vi "Send 2D image to FPGA.vi"(7 "picture":picture, 8 "error in":errorcluster, 11 "FPGA VI Reference Out":T1) -> (0 "error out":errorcluster, 3 "FPGA VI Reference Out 2":T1)   [LabVIEW 2019]
uses:
  TypeDefs/FPGA Reference.ctl
  <vilib>/Utility/error.llb/Error Cluster From Error Code.vi
  <vilib>/rvi/errors/niLvFpgaAdjustHostInterfaceError.vi
  <vilib>/rvi/interface/nirviMethod/nirviMethod.xnode
  FPGA Bitfiles/adafruitlcdsom_FPGATarget_FPGAMain_K7l+4zj6vFY.lvbitx
  FPGA Main.vi
  <vilib>/FPGAPlugInAG/sbRIO-9651/niLvFpga_WriteFifo_sbRIO-9651.vi
  <vilib>/rvi/errors/niLvFpgaMergeErrorWithErrorCode.vi
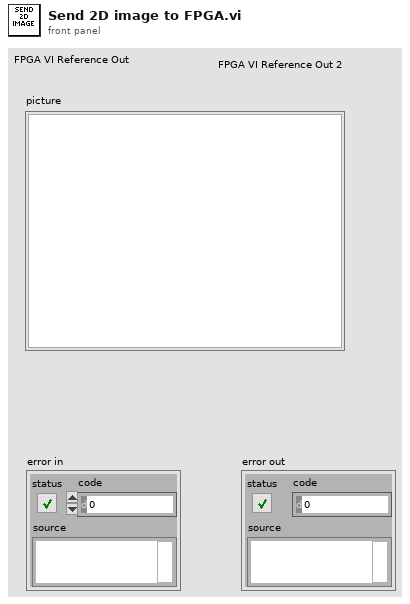
[diagram p1: front panel]
types:
  T1 = typedef "FPGA Reference.ctl" = refnum<k20>
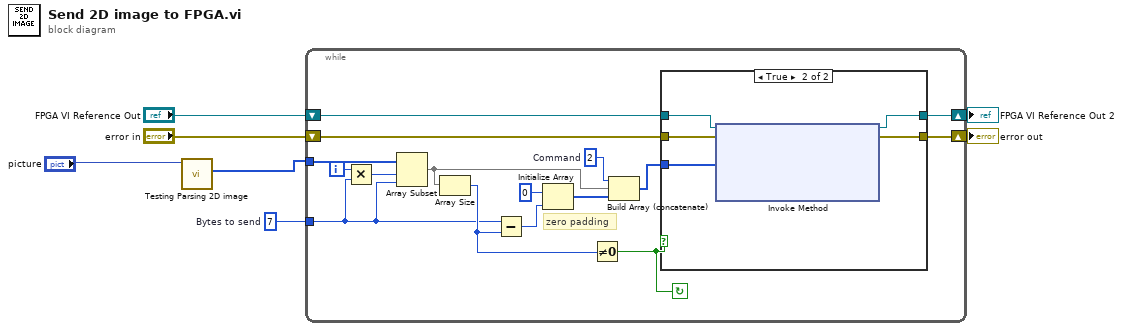
[diagram p0: block diagram]
diagram:
  w4 = 7  # Bytes to send
  n1 = call "Testing Parsing 2D image.vi"("2D Picture"="picture") -> ("output array"=w1:u16[])  [unwired: 9 in, 1 out]
  n2 = while {
    shift-right: [w22] -> w6
    shift-left: "FPGA VI Reference Out" -> [w23]
    shift-right: [w21] -> w5
    shift-left: "error in" -> [w20]
    tunnel: w1 -> [w17]
    tunnel: w4 -> [w8]
    i -> [w16]
    stop <- w11 continue-if-true
    w19 = u16 2  # Command
    # "zero padding"
    n3 = Multiply(x=w16, y=w8) -> (x*y=w15:i32)
    n4 = Array Subset(array=w17, index=w15, length=w8) -> (w14:u16[])
    n5 = Array Size(array=w14) -> (size(s)=w10:i32)
    n6 = Subtract(x=w8, y=w10) -> (x-y=w9:i32)
    n7 = Initialize Array(u16 0 ("X"), w9) -> (w12:u16[])
    n8 = Not Equal To 0?(x=w10) -> (x != 0?=w11:bool)
    n9 = Build Array (concatenate)(w19, w14, w12) -> (w18:u16[])
    n10 = case shown="True" w11 {
      tunnel: w23 -> [w25 w30]
      tunnel: [w25 w29] -> w22
      tunnel: [w24 w28] -> w21
      tunnel: w20 -> [w24 w27]
      tunnel: w18 -> [_ w26]
      frame False {
      }
      frame True {
        n11 = xnode "Invoke Method"("FPGA VI Reference In"=w30, "error in"=w27, "Data"=w26) -> ("FPGA VI Reference Out"=w29:T1, "error out"=w28:errorcluster)  [unwired: 1 in, 1 out]
      }
    }
  }
  "FPGA VI Reference Out 2" <- w6
  "error out" <- w5
